vi "Update Cursors from Measurement Cursor Configuration.vi"(11 "State in":T1={"Graph Visible Items"={"Plot Legend"=FALSE, "Scale Legend"=FALSE, "Graph Palette"=FALSE, "Cursor Legend"=FALSE, "X Scrollbar"=FALSE}, "View Table"=FALSE, "Table Visible Items"={"Vertical Scrollbar"=FALSE, "Horizontal Scrollbar"=FALSE, "Row Headers"=FALSE, "Column Headers"=FALSE, "Vertical Lines"=FALSE, "Horizontal Lines"=FALSE}, "Header Font"={"Font Name"="", "Size"=0, "Bold"=FALSE, "Italic"=FALSE, "Underline"=FALSE, "Strikeout"=FALSE, "Color"=0}, "Cell Font"={"Font Name"="", "Size"=0, "Bold"=FALSE, "Italic"=FALSE, "Underline"=FALSE, "Strikeout"=FALSE, "Color"=0}, "Description and Tip..."={"Description"="", "Tip"=""}, "Moveable Splitter Position"=0, "Measurement Cursor Configuration"={"relative to t0"={"enable relative time"=FALSE, "Relative times (DT)"=[], "color"=0}, "range"={"enable range"=FALSE, "T1"=0.0, "T2"=0.0, "Fixed interval (T2-T1)"=0.0, "T1 color"=0, "T2 color"=0, "enable shading"=FALSE}, "periodic"={"enable periodic"=FALSE, "First event (E1)"=0.0, "Number events (Ei)"=0, "Event spacing (s)"=0.0, "First color"=0, "Events color"=0}, "absolute timestamp"={"enable absolute"=FALSE, "Timestamps (TS)"=[], "color"=0}}, "X Increment"=0.0, "X Scale"={"Label Visible"=FALSE, "Label Text"="", "Time Mode"=enum."Relative", "Format String"=""}, "Y Scale"={"Label Visible"=FALSE, "Label Text"="", "Scaling"=enum."Engineering Units", "Format String"=""}, "Colors"={"background"=16777215, "major grid"=8355711, "minor grid"=12632256, "font"=0}, "Cursors"={"List"=[], "Tags"=[]}, "Plots"=[], "Plot Color Wheel"=[3381759, 32768, 982784, 4375295, 13827953, 13457919, 16757522, 4343295, 16728758, 12095254], "registered user events"=variant} caption="State") -> (3 "State out":T1={"Graph Visible Items"={"Plot Legend"=FALSE, "Scale Legend"=FALSE, "Graph Palette"=FALSE, "Cursor Legend"=FALSE, "X Scrollbar"=FALSE}, "View Table"=FALSE, "Table Visible Items"={"Vertical Scrollbar"=FALSE, "Horizontal Scrollbar"=FALSE, "Row Headers"=FALSE, "Column Headers"=FALSE, "Vertical Lines"=FALSE, "Horizontal Lines"=FALSE}, "Header Font"={"Font Name"="", "Size"=0, "Bold"=FALSE, "Italic"=FALSE, "Underline"=FALSE, "Strikeout"=FALSE, "Color"=0}, "Cell Font"={"Font Name"="", "Size"=0, "Bold"=FALSE, "Italic"=FALSE, "Underline"=FALSE, "Strikeout"=FALSE, "Color"=0}, "Description and Tip..."={"Description"="", "Tip"=""}, "Moveable Splitter Position"=0, "Measurement Cursor Configuration"={"relative to t0"={"enable relative time"=FALSE, "Relative times (DT)"=[], "color"=0}, "range"={"enable range"=FALSE, "T1"=0.0, "T2"=0.0, "Fixed interval (T2-T1)"=0.0, "T1 color"=0, "T2 color"=0, "enable shading"=FALSE}, "periodic"={"enable periodic"=FALSE, "First event (E1)"=0.0, "Number events (Ei)"=0, "Event spacing (s)"=0.0, "First color"=0, "Events color"=0}, "absolute timestamp"={"enable absolute"=FALSE, "Timestamps (TS)"=[], "color"=0}}, "X Increment"=0.0, "X Scale"={"Label Visible"=FALSE, "Label Text"="", "Time Mode"=enum."Relative", "Format String"=""}, "Y Scale"={"Label Visible"=FALSE, "Label Text"="", "Scaling"=enum."Engineering Units", "Format String"=""}, "Colors"={"background"=16777215, "major grid"=8355711, "minor grid"=12632256, "font"=0}, "Cursors"={"List"=[], "Tags"=[]}, "Plots"=[], "Plot Color Wheel"=[3381759, 32768, 982784, 4375295, 13827953, 13457919, 16757522, 4343295, 16728758, 12095254], "registered user events"=variant} caption="State")   [LabVIEW 2017, in "Waveforms with Cursors.xctl"]
doc: "Set cursor attributes. Set cursor list for graph. Add cursors [{ref,tags}] to display state."
uses:
  <vilib>/addons/_XControls/Waveforms with Cursors/Waveforms with Cursors.xctl
  <vilib>/addons/_XControls/Waveforms with Cursors/Controls/State.ctl
  <vilib>/Utility/miscctls.llb/LVFontTypeDef.ctl
  <vilib>/addons/_XControls/Waveforms with Cursors/Controls/Waveform Cursor Configuration.ctl
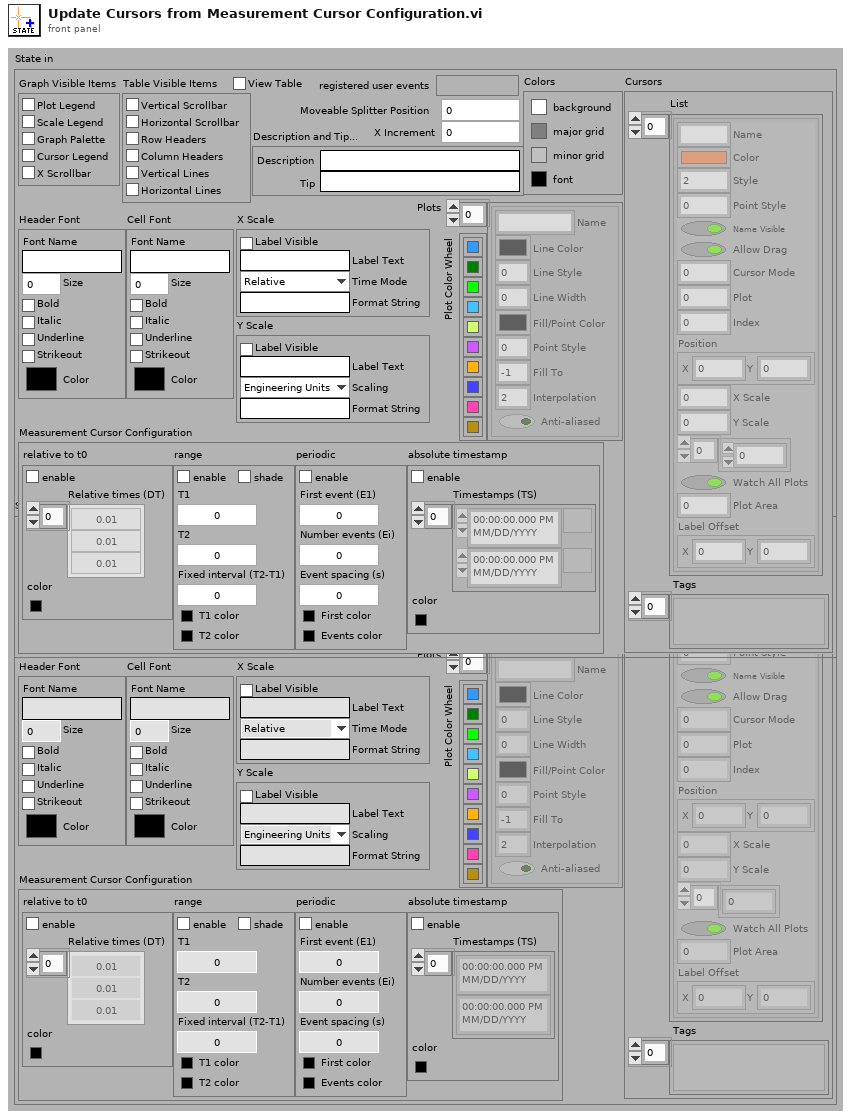
[diagram p1: front panel]
types:
  T1 = typedef "Waveforms with Cursors.xctl/State.ctl" = cluster{"Graph Visible Items":cluster{"Plot Legend":bool, "Scale Legend":bool, "Graph Palette":bool, "Cursor Legend":bool, "X Scrollbar":bool}, "View Table":bool, "Table Visible Items":cluster{"Vertical Scrollbar":bool, "Horizontal Scrollbar":bool, "Row Headers":bool, "Column Headers":bool, "Vertical Lines":bool, "Horizontal Lines":bool}, "Header Font":T2, "Cell Font":T2, "Description and Tip...":cluster{"Description":string, "Tip":string}, "Moveable Splitter Position":i32, "Measurement Cursor Configuration":T3, "X Increment":dbl, "X Scale":cluster{"Label Visible":bool, "Label Text":string, "Time Mode":enum16{"Relative", "Absolute"}, "Format String":string}, "Y Scale":cluster{"Label Visible":bool, "Label Text":string, "Scaling":enum16{"Engineering Units", "Voltage"}, "Format String":string}, "Colors":cluster{"background":u32, "major grid":u32, "minor grid":u32, "font":u32}, "Cursors":cluster{"List":cluster{"Name":string, "Color":u32, "Style":i32, "Point Style":u8, "Name Visible":bool, "Allow Drag":bool, "Cursor Mode":u32, "Plot":i32, "Index":i32, "Position":cluster{"X":dbl, "Y":dbl}, "X Scale":u32, "Y Scale":u32, "Watch Plots":i32[], "Watch All Plots":bool, "Plot Area":i32, "Label Offset":cluster{"X":dbl, "Y":dbl}}[], "Tags":variant[]}, "Plots":cluster{"Name":string, "Line Color":u32, "Line Style":u8, "Line Width":u8, "Fill/Point Color":u32, "Point Style":u8, "Fill To":i16, "Interpolation":u8, "Anti-aliased":bool}[], "Plot Color Wheel":u32[], "registered user events":variant}
  T2 = typedef "LVFontTypeDef.ctl" = cluster{"Font Name":string, "Size":u16, "Bold":bool, "Italic":bool, "Underline":bool, "Strikeout":bool, "Color":u32}
  T3 = typedef "Waveforms with Cursors.xctl/Waveform Cursor Configuration.ctl" = cluster{"relative to t0":cluster{"enable relative time":bool, "Relative times (DT)":dbl[], "color":u32}, "range":cluster{"enable range":bool, "T1":dbl, "T2":dbl, "Fixed interval (T2-T1)":dbl, "T1 color":u32, "T2 color":u32, "enable shading":bool}, "periodic":cluster{"enable periodic":bool, "First event (E1)":dbl, "Number events (Ei)":i32, "Event spacing (s)":dbl, "First color":u32, "Events color":u32}, "absolute timestamp":cluster{"enable absolute":bool, "Timestamps (TS)":timestamp[], "color":u32}}
  T4 = cluster{"Name":string, "Color":u32, "Style":i32, "Point Style":u8, "Name Visible":bool, "Allow Drag":bool, "Cursor Mode":u32, "Plot":i32, "Index":i32, "Position":cluster{"X":dbl, "Y":dbl}, "X Scale":u32, "Y Scale":u32, "Watch Plots":i32[], "Watch All Plots":bool, "Plot Area":i32, "Label Offset":cluster{"X":dbl, "Y":dbl}}
  T5 = cluster{"Name":string, "Color":u32, "Style":i32, "Point Style":u8, "Name Visible":bool, "Allow Drag":bool, "Cursor Mode":u32, "Plot":i32, "Index":i32, "Position":cluster{"X":dbl, "Y":dbl}, "X Scale":u32, "Y Scale":u32, "Watch Plots":i32[], "Watch All Plots":bool, "Plot Area":i32, "Label Offset":cluster{"X":dbl, "Y":dbl}}[]
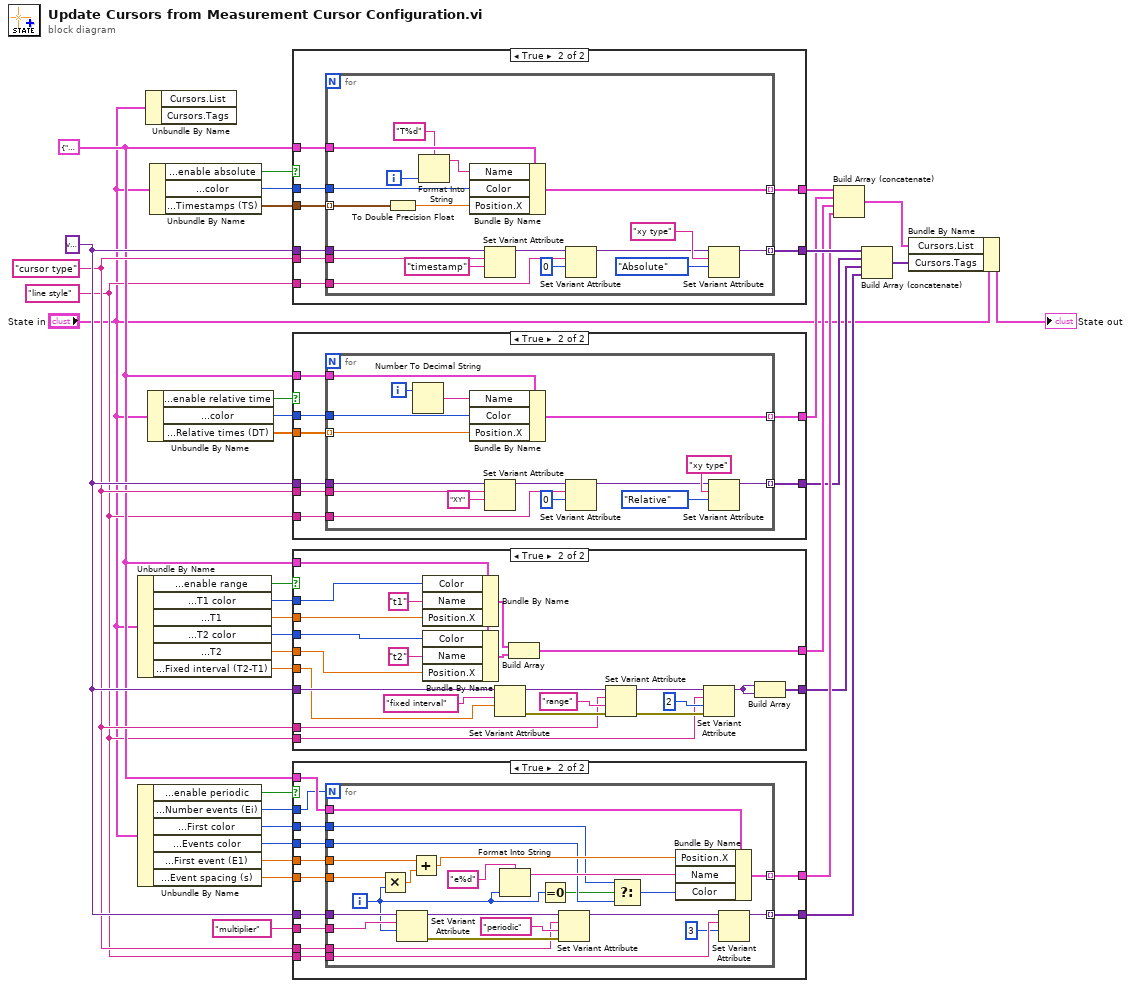
[diagram p0: block diagram]
diagram:
  w14 = "cursor type"
  w2 = "line style"
  w15 = variant ("tags")
  w13 = T4 {"Name"="", "Color"=16744512, "Style"=2, "Point Style"=0, "Name Visible"=TRUE, "Allow Drag"=TRUE, "Cursor Mode"=0, "Plot"=0, "Index"=0, "Position"={"X"=0.0, "Y"=0.0}, "X Scale"=0, "Y Scale"=0, "Watch Plots"=[], "Watch All Plots"=TRUE, "Plot Area"=0, "Label Offset"={"X"=0.0, "Y"=0.0}}
  n1 = Unbundle By Name("State in") -> ("Measurement Cursor Configuration.range.enable range"=w34:bool, "Measurement Cursor Configuration.range.T1 color"=w30:u32, "Measurement Cursor Configuration.range.T1"=w31:dbl, "Measurement Cursor Configuration.range.T2 color"=w29:u32, "Measurement Cursor Configuration.range.T2"=w33:dbl, "Measurement Cursor Configuration.range.Fixed interval (T2-T1)"=w32:dbl)
  n2 = Unbundle By Name("State in") -> ("Measurement Cursor Configuration.periodic.enable periodic"=w28:bool, "Measurement Cursor Configuration.periodic.Number events (Ei)"=w19:i32, "Measurement Cursor Configuration.periodic.First color"=w25:u32, "Measurement Cursor Configuration.periodic.Events color"=w24:u32, "Measurement Cursor Configuration.periodic.First event (E1)"=w26:dbl, "Measurement Cursor Configuration.periodic.Event spacing (s)"=w27:dbl)
  n3 = Unbundle By Name("State in") -> ()  [unwired: 2 out]
  n4 = Unbundle By Name("State in") -> ("Measurement Cursor Configuration.relative to t0.enable relative time"=w22:bool, "Measurement Cursor Configuration.relative to t0.color"=w21:u32, "Measurement Cursor Configuration.relative to t0.Relative times (DT)"=w23:dbl[])
  n5 = Unbundle By Name("State in") -> ("Measurement Cursor Configuration.absolute timestamp.enable absolute"=w18:bool, "Measurement Cursor Configuration.absolute timestamp.color"=w17:u32, "Measurement Cursor Configuration.absolute timestamp.Timestamps (TS)"=w16:timestamp[])
  n6 = case shown="True" w18 {
    tunnel: w13 -> [_ w43]
    tunnel: w16 -> [_ w42]
    tunnel: [_ w41] -> w12
    tunnel: w15 -> [_ w40]
    tunnel: [_ w39] -> w11
    tunnel: w17 -> [_ w38]
    tunnel: w14 -> [_ w37]
    tunnel: w2 -> [_ w36]
    frame False {
    }
    frame True {
      n7 = for {
        tunnel: w43 -> [w55]
        tunnel: w42 -> [w60] mode=indexing
        tunnel: [w61] -> w41 mode=indexing
        tunnel: w40 -> [w58]
        tunnel: [w54] -> w39 mode=indexing
        tunnel: w38 -> [w47]
        tunnel: w37 -> [w52]
        tunnel: w36 -> [w51]
        i -> [w46]
        n8 = To Double Precision Float(number=w60) -> (double precision float=w48:dbl)
        n9 = Format Into String(format string="T%d", w46) -> (resulting string=w44:string)  [unwired: 2 in, 1 out]
        n10 = Bundle By Name(cluster=w55, "Name"=w44, "Color"=w47, "Position.X"=w48) -> (w61:T4)
        n11 = Set Variant Attribute(Variant=w58, name=w52, value="timestamp") -> (Variant out=w57:variant)  [unwired: 1 in, 2 out]
        n12 = Set Variant Attribute(Variant=w57, name=w51, value=u8 0 ("Line Style")) -> (Variant out=w50:variant)  [unwired: 1 in, 2 out]
        n13 = Set Variant Attribute(Variant=w50, name="xy type", value=enum16{"Relative", "Absolute"}."Absolute" ("X Scale.Time Mode")) -> (Variant out=w54:variant)  [unwired: 1 in, 2 out]
      }
    }
  }
  n14 = case shown="True" w22 {
    tunnel: w13 -> [_ w69]
    tunnel: w23 -> [_ w68]
    tunnel: [_ w67] -> w10
    tunnel: w15 -> [_ w66]
    tunnel: [_ w65] -> w7
    tunnel: w21 -> [_ w64]
    tunnel: w14 -> [_ w63]
    tunnel: w2 -> [_ w62]
    frame False {
    }
    frame True {
      n15 = for {
        tunnel: w69 -> [w78]
        tunnel: w68 -> [w83] mode=indexing
        tunnel: [w85] -> w67 mode=indexing
        tunnel: w66 -> [w81]
        tunnel: [w77] -> w65 mode=indexing
        tunnel: w64 -> [w75]
        tunnel: w63 -> [w74]
        tunnel: w62 -> [w73]
        i -> [w84]
        n16 = Number To Decimal String(number=w84) -> (decimal integer string=w72:string)  [unwired: 1 in]
        n17 = Bundle By Name(cluster=w78, "Name"=w72, "Color"=w75, "Position.X"=w83) -> (w85:T4)
        n18 = Set Variant Attribute(Variant=w81, name=w74, value="XY") -> (Variant out=w80:variant)  [unwired: 1 in, 2 out]
        n19 = Set Variant Attribute(Variant=w80, name=w73, value=u8 0 ("Line Style")) -> (Variant out=w71:variant)  [unwired: 1 in, 2 out]
        n20 = Set Variant Attribute(Variant=w71, name="xy type", value=enum16{"Relative", "Absolute"}."Relative" ("X Scale.Time Mode")) -> (Variant out=w77:variant)  [unwired: 1 in, 2 out]
      }
    }
  }
  n21 = case shown="True" w34 {
    tunnel: w33 -> [_ w105]
    tunnel: w32 -> [_ w99]
    tunnel: w13 -> [_ w94]
    tunnel: w31 -> [_ w106]
    tunnel: [_ w103] -> w9
    tunnel: w15 -> [_ w101]
    tunnel: [_ w98] -> w6
    tunnel: w30 -> [_ w93]
    tunnel: w29 -> [_ w92]
    tunnel: w14 -> [_ w87]
    tunnel: w2 -> [_ w86]
    frame False {
    }
    frame True {
      n22 = Bundle By Name(cluster=w94, "Color"=w93, "Name"="t1" ("format string"), "Position.X"=w106) -> (w102:T4)
      n23 = Bundle By Name(cluster=w94, "Color"=w92, "Name"="t2", "Position.X"=w105) -> (w104:T4)
      n24 = Set Variant Attribute(Variant=w101, name="fixed interval", value=w99) -> (Variant out=w96:variant, error out=w97:errorcluster)  [unwired: 1 in, 1 out]
      n25 = Build Array(w102, w104) -> (w103:T5)
      n26 = Set Variant Attribute(Variant=w96, name=w87, value="range", error in=w97) -> (Variant out=w91:variant, error out=w89:errorcluster)  [unwired: 1 out]
      n27 = Set Variant Attribute(Variant=w91, name=w86, value=u8 2 ("Line Style"), error in=w89) -> (Variant out=w90:variant)  [unwired: 2 out]
      n28 = Build Array(w90, w90) -> (w98:variant[])
    }
  }
  n29 = case shown="True" w28 {
    tunnel: w27 -> [_ w118]
    tunnel: w19 -> [_ w109]
    tunnel: w13 -> [_ w120]
    tunnel: w26 -> [_ w117]
    tunnel: [_ w119] -> w8
    tunnel: w15 -> [_ w116]
    tunnel: [_ w115] -> w5
    tunnel: w25 -> [_ w114]
    tunnel: w24 -> [_ w113]
    tunnel: "multiplier" -> [_ w112]
    tunnel: w2 -> [_ w111]
    tunnel: w14 -> [_ w110]
    frame False {
    }
    frame True {
      n30 = for {
        N: w109 -> [_]
        tunnel: w120 -> [w132]
        tunnel: [w142] -> w119 mode=indexing
        tunnel: w118 -> [w141]
        tunnel: w117 -> [w140]
        tunnel: w112 -> [w137]
        tunnel: w116 -> [w136]
        tunnel: [w130] -> w115 mode=indexing
        tunnel: w114 -> [w125]
        tunnel: w113 -> [w124]
        tunnel: w111 -> [w128]
        tunnel: w110 -> [w127]
        i -> [w121]
        n31 = Multiply(x=w141, y=w121) -> (x*y=w139:dbl)
        n32 = Set Variant Attribute(Variant=w136, name=w137, value=w121) -> (Variant out=w133:variant, error out=w134:errorcluster)  [unwired: 1 in, 1 out]
        n33 = Add(x=w140, y=w139) -> (x+y=w138:dbl)
        n34 = Format Into String(format string="e%d", w121) -> (resulting string=w143:string)  [unwired: 2 in, 1 out]
        n35 = Equal To 0?(x=w121) -> (x = 0?=w122:bool)
        n36 = Set Variant Attribute(Variant=w133, name=w127, value="periodic", error in=w134) -> (Variant out=w131:variant)  [unwired: 2 out]
        n37 = Select(t=w125, s=w122, f=w124) -> (s? t:f=w123:u32)
        n38 = Bundle By Name(cluster=w132, "Position.X"=w138, "Name"=w143, "Color"=w123) -> (w142:T4)
        n39 = Set Variant Attribute(Variant=w131, name=w128, value=u8 3 ("Line Style")) -> (Variant out=w130:variant)  [unwired: 1 in, 2 out]
      }
    }
  }
  n40 = Build Array (concatenate)(w12, w10, w9, w8) -> (w3:T5)
  n41 = Build Array (concatenate)(w11, w7, w6, w5) -> (w4:variant[])
  n42 = Bundle By Name(cluster="State in", "Cursors.List"=w3, "Cursors.Tags"=w4) -> (→"State out":T1)
